vi "TestSubtract.vi"   [LabVIEW 2016, in "SimpleCalculatorTests.lvlib"]
uses:
  SimpleCalculatorTests.lvlib
  APIs/Stimulus/ControlValue/SetValueAuto.vi
  APIs/Assert/AssertControlValue/AlmostEqual.vi
  Drona.lvlib
  <vilib>/addons/_JKI Toolkits/Caraya/classes/Test/Test.lvclass
  APIs/Stimulus/ControlValue/ControlValue.lvlib
  APIs/Assert/AssertControlValue/AssertControlValue.lvlib
panel:
  # "Drona Test Subtract"
types:
  T1 = cluster{"Input 1":dbl, "Input 2":dbl, "Output":dbl}[]
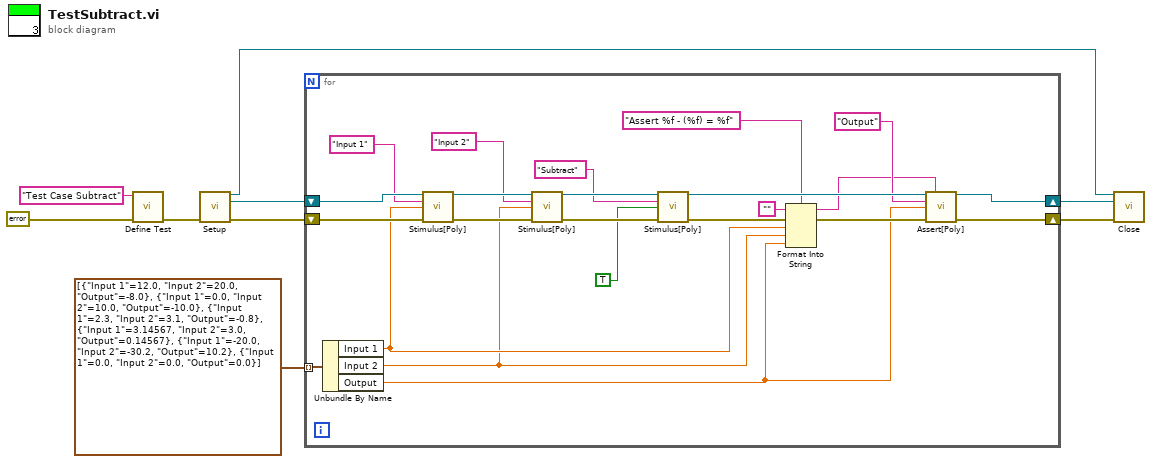
[diagram p0: block diagram]
diagram:
  n1 = call <vilib>:"Define Test.vi"("error in (no error)"=errorcluster {"status"=FALSE, "code"=0, "source"=""} ("error in"), "Label (VI Title)"="Test Case Subtract") -> ("error out"=w3:errorcluster)  [unwired: 9 in]
  n2 = call "Setup.vi"("error in"=w3) -> ("Application Ref"=w7:refnum<vi>, "VI Reference Out"=w9:refnum<vi>, "error out"=w8:errorcluster)  [unwired: 12 in]
  n3 = for {
    shift-right: [w20] -> w4
    shift-left: w9 -> [w32]
    shift-right: [w22] -> w5
    shift-left: w8 -> [w31]
    tunnel: T1 [{"Input 1"=12.0, "Input 2"=20.0, "Output"=-8.0}, {"Input 1"=0.0, "Input 2"=10.0, "Output"=-10.0}, {"Input 1"=2.3, "Input 2"=3.1, "Output"=-0.8}, {"Input 1"=3.14567, "Input 2"=3.0, "Output"=0.14567}, {"Input 1"=-20.0, "Input 2"=-30.2, "Output"=10.2}, {"Input 1"=0.0, "Input 2"=0.0, "Output"=0.0}] -> [w18] mode=indexing
    n4 = Unbundle By Name(w18) -> ("Input 1"=w15:dbl, "Input 2"=w14:dbl, "Output"=w13:dbl)
    n5 = call-poly "Stimulus[Poly].vi"("VI Reference In"=w32, "Control Path"="Input 1", "Value (Signaling)"=w15, "error in"=w31) -> ("VI Reference Out"=w28:refnum<vi>, "error out"=w29:errorcluster)  [unwired: 10 in]
    n6 = call-poly "Stimulus[Poly].vi"("VI Reference In"=w28, "Control Path"="Input 2", "Value (Signaling)"=w14, "error in"=w29) -> ("VI Reference Out"=w26:refnum<vi>, "error out"=w25:errorcluster)  [unwired: 10 in]
    n7 = call-poly "Stimulus[Poly].vi"("VI Reference In"=w26, "Control Path"="Subtract", "Value (Signaling)"=TRUE, "error in"=w25) -> ("VI Reference Out"=w21:refnum<vi>, "error out"=w23:errorcluster)  [unwired: 10 in]
    n8 = Format Into String(format string="Assert %f - (%f) = %f", initial string="", error in=w23, w15, w14, w13) -> (resulting string=w12:string, error out=w17:errorcluster)
    n9 = call-poly "Assert[Poly].vi"("VI Reference In"=w21, "Label"=w12, "Control Path"="Output", "Control Value"=w13, "Error In"=w17) -> ("VI Reference Out"=w20:refnum<vi>, "Error Out"=w22:errorcluster)  [unwired: 9 in]
  }
  n10 = call "Close.vi"("Application Ref"=w7, "VI Reference Out"=w4, "error in"=w5) -> ()  [unwired: 12 in, 1 out]
